vi "Single GPIO.vi"() -> ()   [LabVIEW 2023, in "CTI-Visa-Scratchpad.lvlib"]
uses:
  CTI-Visa-Scratchpad.lvlib
  CTI-Visa/Digital Direction.ctl
  CTI-Visa/CTI-Visa.lvlib
panel:
  in  "GPIO":i32=2
  out "Readback":bool
  in  "Control":bool
  in  "Port":refnum<visa-resource-name>="COM3"
  in  "stop":bool
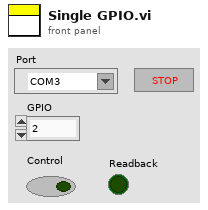
[diagram p1: front panel]
types:
  T1 = typedef "CTI-Visa.lvlib/Digital Direction.ctl" = enum16{"In", "Out"}
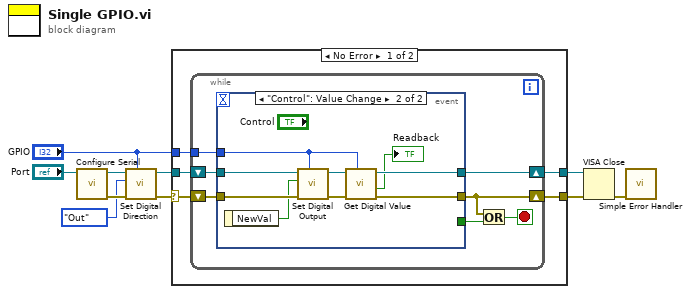
[diagram p0: block diagram]
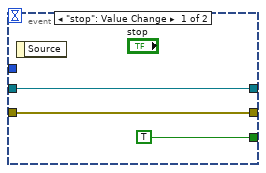
[diagram p2: hidden frame]
diagram:
  n1 = call "Configure Serial.vi"("VISA resource name in"="Port") -> ("error out"=w8:errorcluster, "VISA resource name"=w9:refnum<visa-resource-name>)  [unwired: 9 in]
  n2 = call "Set Digital Direction.vi"("GPIO"="GPIO", "error in (no error)"=w8, "Direction"=Digital_Direction."Out", "VISA resource name in"=w9) -> ("error out"=w6:errorcluster, "VISA resource name"=w7:refnum<visa-resource-name>)  [unwired: 6 in]
  n3 = case shown="No Error" w6 {
    selector: w6 -> [w14 w35]
    tunnel: w7 -> [w15 w36]
    tunnel: [w13 w36] -> w5
    tunnel: [w12 w35] -> w4
    tunnel: "GPIO" -> [w11 _]
    frame No Error {
      n4 = while {
        shift-right: [w20] -> w13
        shift-left: w15 -> [w22]
        shift-right: [w19] -> w12
        shift-left: w14 -> [w21]
        tunnel: w11 -> [w16]
        stop <- w18 stop-if-true
        n5 = event shown="[1] \"Control\": Value Change" {
          selector: _ -> [_ _]
          dyn-events: _ -> [_ _]
          timeout: _ -> [_ _]
          tunnel: w22 -> [w25 w34]
          tunnel: w21 -> [w24 w33]
          tunnel: [w25 w32] -> w20
          tunnel: [w24 w31] -> w19
          tunnel: [TRUE _] -> w17
          tunnel: w16 -> [_ w27]
          event "stop": Value Change {
            n6 = event-data() -> ()  [unwired: 1 in, 1 out]
          }
          event "Control": Value Change {
            n7 = event-data() -> ("NewVal"=w26:bool)  [unwired: 1 in]
            n8 = call "Set Digital Output.vi"("GPIO"=w27, "error in (no error)"=w33, "Value"=w26, "VISA resource name in"=w34) -> ("error out"=w29:errorcluster, "VISA resource name"=w30:refnum<visa-resource-name>)  [unwired: 6 in]
            n9 = call "Get Digital Value.vi"("GPIO"=w27, "error in (no error)"=w29, "VISA resource name in"=w30) -> ("error out"=w31:errorcluster, "Value"=→"Readback":bool, "VISA resource name"=w32:refnum<visa-resource-name>)  [unwired: 6 in]
          }
        }
        n10 = Or(x=w19, y=w17) -> (x .or. y?=w18:bool)
      }
    }
    frame Error {
    }
  }
  n11 = VISA Close(VISA resource name=w5, error in (no error)=w4) -> (error out=w3:errorcluster)
  n12 = call <vilib>:"Simple Error Handler.vi"("error in (no error)"=w3) -> ()  [unwired: 4 in, 5 out]
